vi "SetFunctionParams.vi"(8 "error in (no error)":errorcluster, 10 "FunctionParams":variant, 11 "PmuAnalysis in":refnum<class "PmuAnalysis.lvclass">) -> (0 "error out":errorcluster, 3 "PmuAnalysis out":refnum<class "PmuAnalysis.lvclass">)   [LabVIEW 2018, in "AnalysisPlugins.lvlib" / "PmuAnalysis.lvclass"]
uses:
  PmuAnalysis.lvclass
  PmuAnalysis.lvclass/PmuAnalysis.ctl
  Accessors/Read Function.vi
  Accessors/Write Function.vi
  FGen/MemberClasses/FunctionBaseClass/FunctionBase.lvclass
panel:
  # "Not all analysis plugins will\nhave function classes"
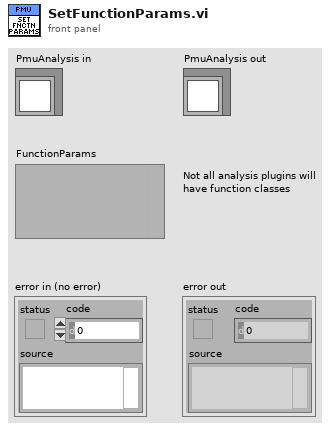
[diagram p1: front panel]
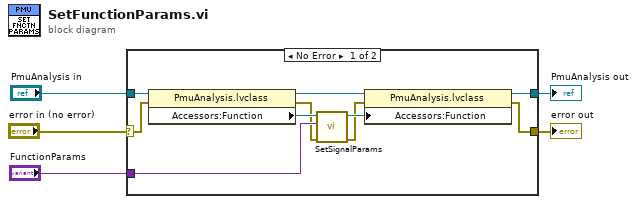
[diagram p0: block diagram]
diagram:
  n1 = case shown="No Error" "error in (no error)" {
    selector: "error in (no error)" -> [w13 w17]
    tunnel: "PmuAnalysis in" -> [w15 w16]
    tunnel: "FunctionParams" -> [w12 _]
    tunnel: [w6 w17] -> w1
    tunnel: [w7 w16] -> w2
    frame No Error {
      n2 = property class="PmuAnalysis.lvclass"(reference=w15, error in=w13) -> (reference out=w10:refnum<class "PmuAnalysis.lvclass">, error out=w11:errorcluster, "Accessors:Function"=w14:refnum<class "FunctionBase.lvclass">)
      n3 = call-dynamic "SetSignalParams.vi"("error in (no error)"=w11, "Variant"=w12, "FunctionBase in"=w14) -> ("error out"=w8:errorcluster, "FunctionBase out"=w9:refnum<class "FunctionBase.lvclass">)  [unwired: 7 in]
      n4 = property class="PmuAnalysis.lvclass"(reference=w10, error in=w8, "Accessors:Function"=w9) -> (reference out=w7:refnum<class "PmuAnalysis.lvclass">, error out=w6:errorcluster)
    }
    frame Error {
    }
  }
  "error out" <- w1
  "PmuAnalysis out" <- w2
